vi "Initialise_bias_source.vi"(7 "output cluster":T1 {"TimeStamp" format="%.2f"}, 8 "error in (no error)":errorcluster, 9 "Load bias parameters":bool) -> (0 "error out":errorcluster {"code" format="%.0x"}, 1 "Response to Load bias parameters":string, 2 "Response Initialise":string)   [LabVIEW 2020]
uses:
  DataSocketCluster external.ctl
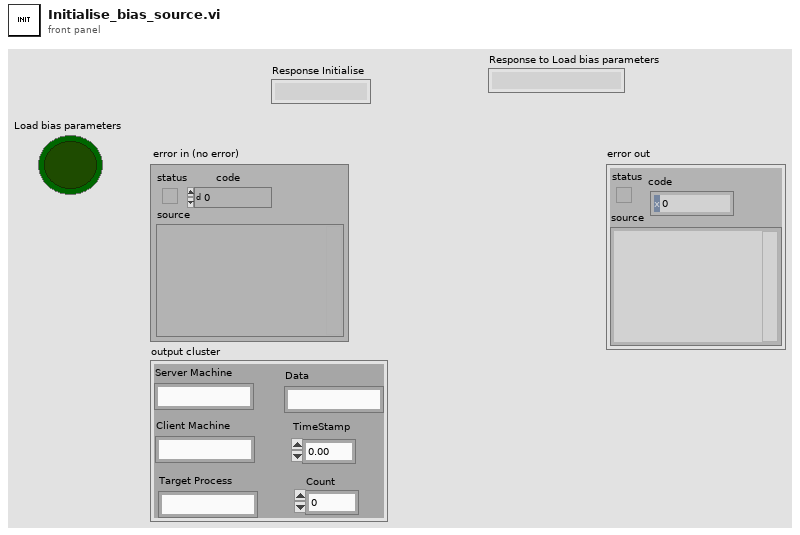
[diagram p1: front panel]
types:
  T1 = typedef "DataSocketCluster external.ctl" = cluster{"Server Machine":string, "Client Machine":string, "Data":string, "TimeStamp":dbl, "Count":i32, "Target Process":string}
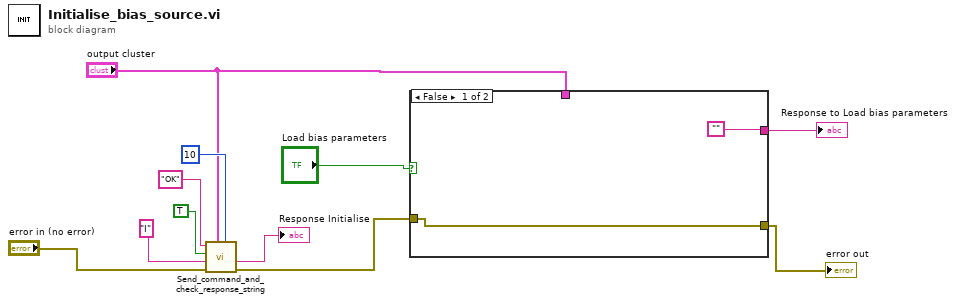
[diagram p0: block diagram]
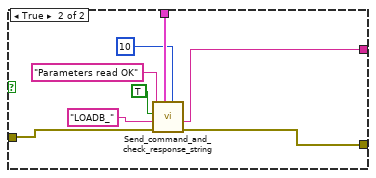
[diagram p2: hidden frame]
diagram:
  n1 = call "Send_command_and_check_response_string.vi"("milliseconds to wait"=u32 10, "output cluster"="output cluster", "error in (no error)"="error in (no error)", "Command"="I", "test response?"=TRUE, "Expected response"="OK" ("Command")) -> ("error IO"=w4:errorcluster, "Return value"=→"Response Initialise":string)  [unwired: 2 in]
  n2 = case shown="False" "Load bias parameters" {
    tunnel: w4 -> [w13 w21]
    tunnel: [w13 w20] -> w3
    tunnel: "output cluster" -> [_ w19]
    tunnel: ["" w14] -> w1
    frame False {
    }
    frame True {
      n3 = call "Send_command_and_check_response_string.vi"("milliseconds to wait"=u32 10, "output cluster"=w19, "error in (no error)"=w21, "Command"="LOADB_", "test response?"=TRUE, "Expected response"="Parameters read OK" ("Command")) -> ("error IO"=w20:errorcluster, "Return value"=w14:string)  [unwired: 2 in]
    }
  }
  "error out" <- w3
  "Response to Load bias parameters" <- w1
